vi "Win32-Move Window To Back.vi"(8 "error in (no error)":errorcluster, 11 "hWnd":i32) -> (0 "error out":errorcluster)   [LabVIEW 2020]
doc: "Uses Windows API to force panel to stay on top of all other windows."
uses:
  user32.dll
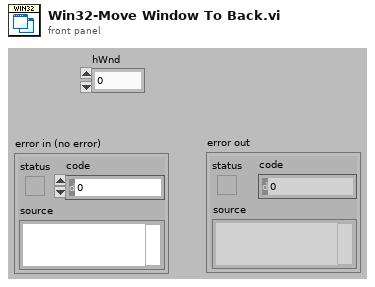
[diagram p1: front panel]
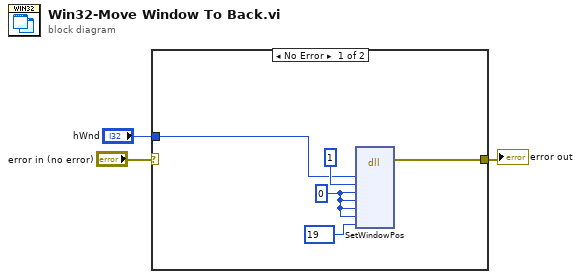
[diagram p0: block diagram]
diagram:
  n1 = case shown="No Error" "error in (no error)" {
    selector: "error in (no error)" -> [_ w9]
    tunnel: [w5 w9] -> w3
    tunnel: "hWnd" -> [w4 _]
    frame No Error {
      w8 = 0 ("X")
      n2 = dll-call lib="user32.dll" fn="SetWindowPos"("hWnd"=w4, "hWndInsertAfter"=1, "X"=w8, "Y"=w8, "cx"=w8, "cy"=w8, "uFlags"=u32 19) -> (error out=w5:errorcluster)  [unwired: 10 in, 2 out]
    }
    frame Error {
    }
  }
  "error out" <- w3
